vi "Unsubscribe.vi"(8 "error in (no error)":errorcluster, 10 "Unsubscriber ID":string, 11 "IViewModel in":refnum<class "IViewModel.lvclass">) -> (0 "error out":errorcluster, 3 "IViewModel out":refnum<class "IViewModel.lvclass">)   [LabVIEW 2015, in "IViewModel.lvlib" / "IViewModel.lvclass"]
doc: "<License>\nCopyright © 2017 Composed Systems, LLC | All rights reserved\nwww.composed.io\n\nAuthor: Ethan Stern <ethan.stern@composed.io>\n\nThis software is provided \"AS IS\" WITHOUT WARRANTIES, either express or implied, AND IS FOR EDUCATIONAL PURPOSES ONLY.\n</License>"
uses:
  IViewModel.lvclass
  IViewModel.lvclass/IViewModel.ctl
  IMediator/IMediator Messages/Unsubscribe Msg/Unsubscribe Msg.lvclass/Unsubscribe Msg.ctl
  <vilib>/ActorFramework/Message Enqueuer/Message Enqueuer.lvclass/Message Enqueuer.ctl
  <vilib>/ActorFramework/Message Enqueuer/Enqueue.vi
  <vilib>/ActorFramework/Message Priority Queue/Priority Enqueue.vi
  IMediator/IMediator Messages/Unsubscribe Msg/Unsubscribe Msg.lvclass
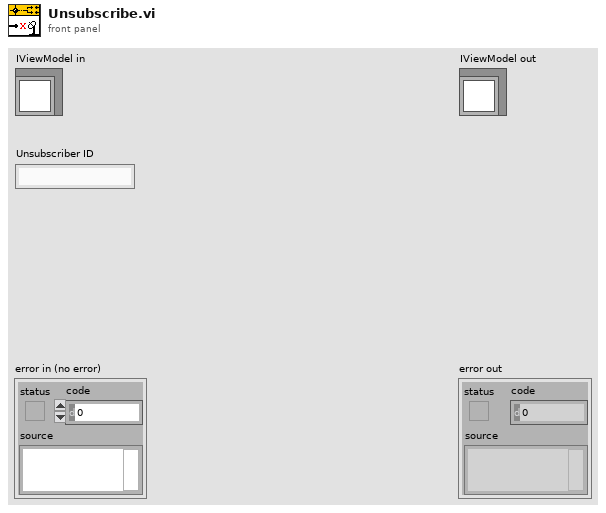
[diagram p1: front panel]
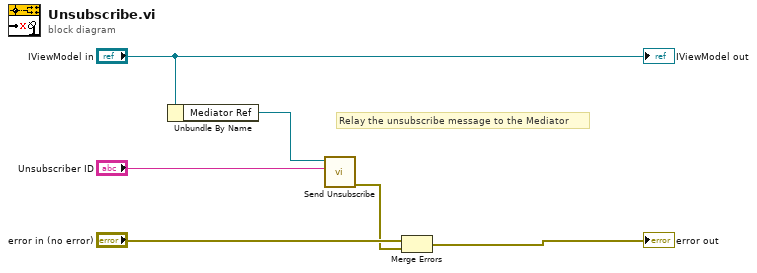
[diagram p0: block diagram]
diagram:
  # "Relay the unsubscribe message to the Mediator"
  n1 = Unbundle By Name("IViewModel in") -> ("Mediator Ref"=w4:refnum<class "Message Enqueuer.lvclass">)
  n2 = call "Send Unsubscribe.vi"("Unsubscriber ID"="Unsubscriber ID", "Message Enqueuer"=w4) -> ("error out"=w1:errorcluster)  [unwired: 8 in, 1 out]
  n3 = Merge Errors("error in (no error)", w1) -> (→"error out":errorcluster)
  "IViewModel out" <- "IViewModel in"
